vi "Servo Open comunication.vi"(8 "error in (no error)":errorcluster, 9 "IP address":T4) -> (0 "error out":errorcluster, 2 "Conections out":T3)   [LabVIEW 2017]
uses:
  <vilib>/addons/eal4LabVIEW/eal4LabVIEW.lvlib
  <vilib>/addons/eal4LabVIEW/ApiLib/Connection control/ealApiConnect_string.vi
  ctl/connections.ctl
  Servo drive module.lvlib
  ctl/Absolute actual position.ctl
  ctl/IP addresses.ctl
  ctl/Axis status.ctl
  ctl/Servo overall status.ctl
panel:
  in  "Overall status":T1
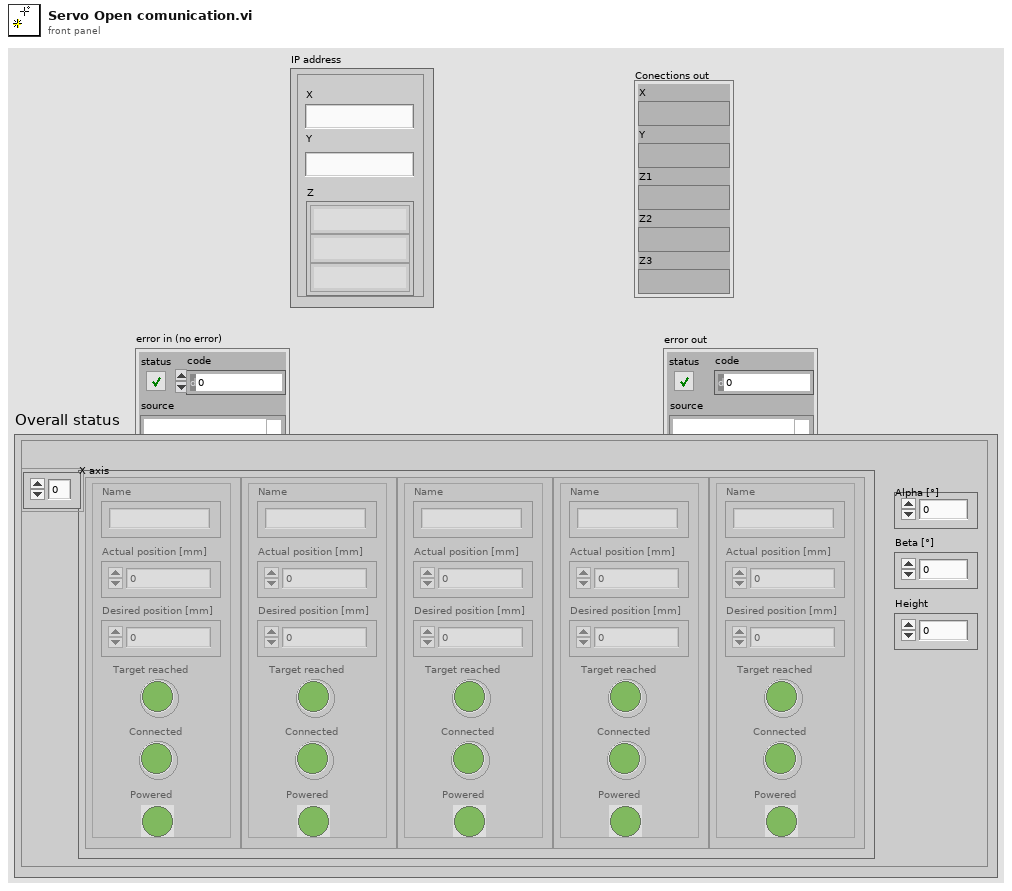
[diagram p1: front panel]
types:
  T1 = typedef "Servo drive module.lvlib/Servo overall status.ctl" = cluster{"X axis":T2[], "Alpha [°]":dbl, "Beta [°]":dbl, "Height":dbl}
  T2 = typedef "Servo drive module.lvlib/Axis status.ctl" = cluster{"Name":string, "Actual position [mm]":dbl, "Desired position [mm]":dbl, "Target reached":bool, "Connected":bool, "Powered":bool}
  T3 = typedef "Servo drive module.lvlib/connections.ctl" = cluster{"X":variant, "Y":variant, "Z1":variant, "Z2":variant, "Z3":variant}
  T4 = typedef "Servo drive module.lvlib/IP addresses.ctl" = cluster{"X":string, "Y":string, "Z":string[]}
  T5 = typedef "Servo drive module.lvlib/Absolute actual position.ctl" = cluster{"X":dbl, "Y":dbl, "Z1":dbl, "Z2":dbl, "Z3":dbl}
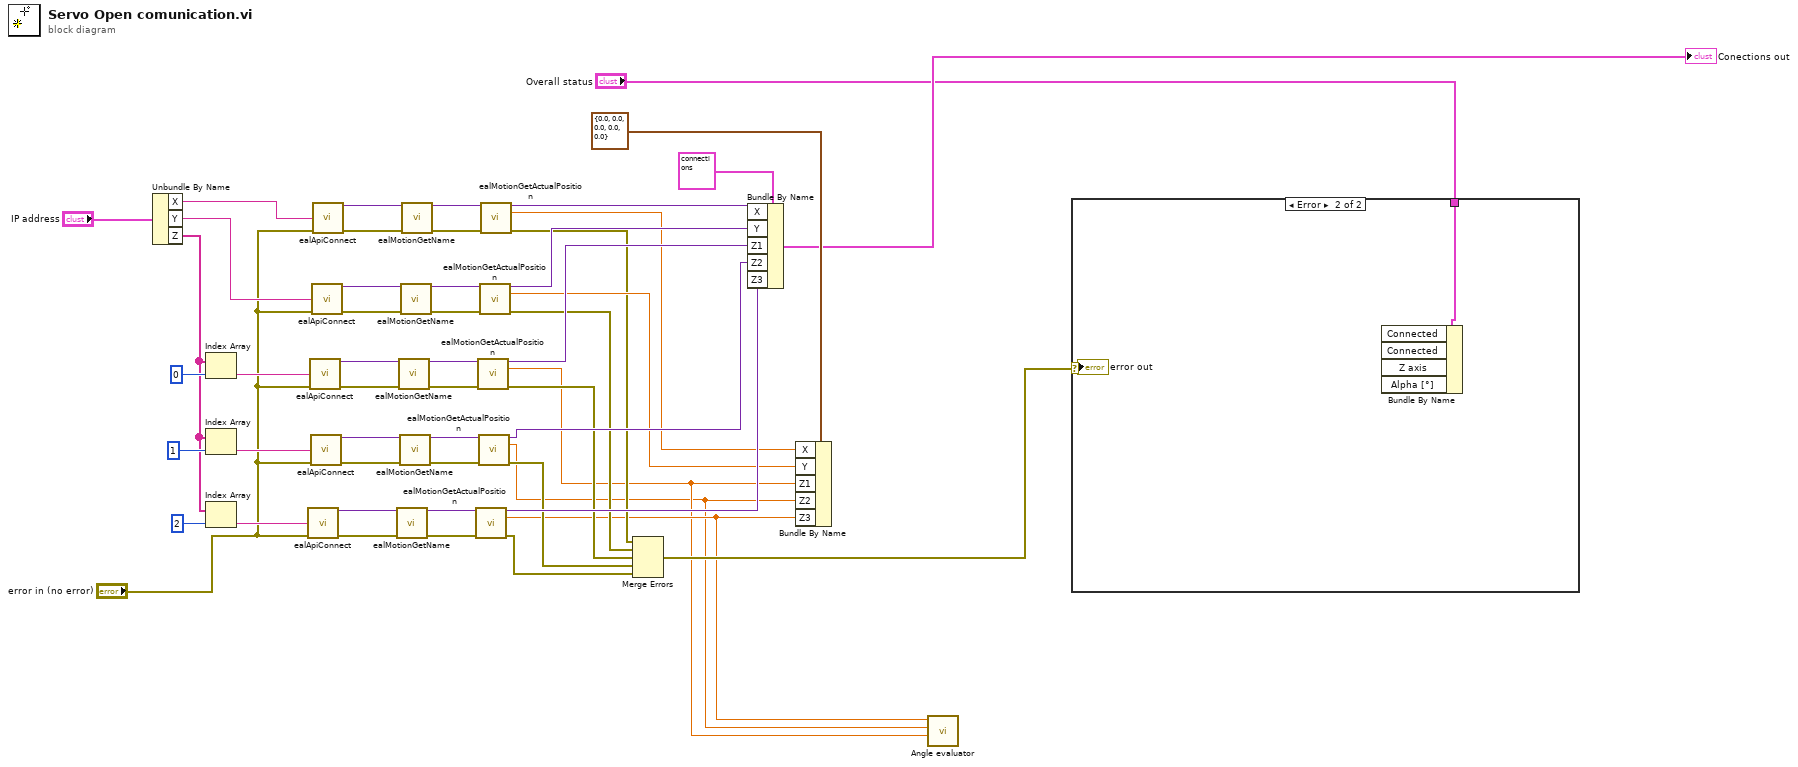
[diagram p0: block diagram]
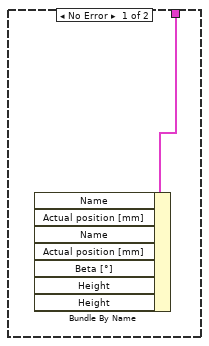
[diagram p2: hidden frame]
diagram:
  n1 = Unbundle By Name("IP address") -> ("X"=w43:string, "Y"=w44:string, "Z"=w45:string[])
  n2 = Index Array(array=w45, index=0) -> (element=w48:string)
  n3 = Index Array(array=w45, index=1) -> (element=w47:string)
  n4 = Index Array(array=w45, index=2) -> (element=w46:string)
  n5 = call-poly <vilib>:"ealApiConnect.vi"("ip address"=w46, "error in (no error)"="error in (no error)") -> ("connection out"=w29:variant, "error out"=w30:errorcluster)  [unwired: 12 in]
  n6 = call-poly <vilib>:"ealApiConnect.vi"("ip address"=w48, "error in (no error)"="error in (no error)") -> ("connection out"=w21:variant, "error out"=w22:errorcluster)  [unwired: 12 in]
  n7 = call-poly <vilib>:"ealApiConnect.vi"("ip address"=w47, "error in (no error)"="error in (no error)") -> ("connection out"=w26:variant, "error out"=w25:errorcluster)  [unwired: 12 in]
  n8 = call-poly <vilib>:"ealApiConnect.vi"("ip address"=w44, "error in (no error)"="error in (no error)") -> ("connection out"=w18:variant, "error out"=w17:errorcluster)  [unwired: 12 in]
  n9 = call-poly <vilib>:"ealApiConnect.vi"("ip address"=w43, "error in (no error)"="error in (no error)") -> ("connection out"=w13:variant, "error out"=w14:errorcluster)  [unwired: 12 in]
  n10 = call <vilib>:"ealMotionGetName.vi"("connection in"=w29, "error in (no error)"=w30) -> ("connection out"=w28:variant, "error out"=w31:errorcluster)  [unwired: 11 in, 1 out]
  n11 = call <vilib>:"ealMotionGetName.vi"("connection in"=w21, "error in (no error)"=w22) -> ("connection out"=w20:variant, "error out"=w23:errorcluster)  [unwired: 11 in, 1 out]
  n12 = call <vilib>:"ealMotionGetName.vi"("connection in"=w26, "error in (no error)"=w25) -> ("connection out"=w27:variant, "error out"=w24:errorcluster)  [unwired: 11 in, 1 out]
  n13 = call <vilib>:"ealMotionGetName.vi"("connection in"=w18, "error in (no error)"=w17) -> ("connection out"=w19:variant, "error out"=w16:errorcluster)  [unwired: 11 in, 1 out]
  n14 = call <vilib>:"ealMotionGetName.vi"("connection in"=w13, "error in (no error)"=w14) -> ("connection out"=w12:variant, "error out"=w15:errorcluster)  [unwired: 11 in, 1 out]
  n15 = call <vilib>:"ealMotionGetActualPosition.vi"("connection in"=w28, "error in (no error)"=w31) -> ("connection out"=w39:variant, "getActualPosition"=w3:dbl, "error out"=w7:errorcluster)  [unwired: 11 in]
  n16 = call <vilib>:"ealMotionGetActualPosition.vi"("connection in"=w20, "error in (no error)"=w23) -> ("connection out"=w37:variant, "getActualPosition"=w2:dbl, "error out"=w9:errorcluster)  [unwired: 11 in]
  n17 = call <vilib>:"ealMotionGetActualPosition.vi"("connection in"=w27, "error in (no error)"=w24) -> ("connection out"=w38:variant, "getActualPosition"=w1:dbl, "error out"=w8:errorcluster)  [unwired: 11 in]
  n18 = call <vilib>:"ealMotionGetActualPosition.vi"("connection in"=w19, "error in (no error)"=w16) -> ("connection out"=w36:variant, "getActualPosition"=w33:dbl, "error out"=w10:errorcluster)  [unwired: 11 in]
  n19 = call <vilib>:"ealMotionGetActualPosition.vi"("connection in"=w12, "error in (no error)"=w15) -> ("connection out"=w35:variant, "getActualPosition"=w32:dbl, "error out"=w11:errorcluster)  [unwired: 11 in]
  n20 = Merge Errors(w11, w10, w9, w8, w7) -> (w5:errorcluster)
  n21 = Bundle By Name(cluster=T3 {"X"=variant, "Y"=variant, "Z1"=variant, "Z2"=variant, "Z3"=variant} ("Conections in"), "X"=w35, "Y"=w36, "Z1"=w37, "Z2"=w38, "Z3"=w39) -> (→"Conections out":T3)
  n22 = Bundle By Name(cluster=T5 {"X"=0.0, "Y"=0.0, "Z1"=0.0, "Z2"=0.0, "Z3"=0.0} ("Actual position in"), "X"=w32, "Y"=w33, "Z1"=w2, "Z2"=w1, "Z3"=w3) -> ()  [unwired: 1 out]
  n23 = call "Angle evaluator.vi"("Position Az"=w2, "Position Bz"=w1, "Position Cz"=w3) -> ()  [unwired: 7 in, 2 out]
  n24 = case shown="Error" w5 {
    selector: w5 -> [_ w54]
    tunnel: "Overall status" -> [w52 w53]
    frame No Error {
      n25 = Bundle By Name(cluster=w52) -> ()  [unwired: 7 in, 1 out]
    }
    frame Error {
      n26 = Bundle By Name(cluster=w53) -> ()  [unwired: 4 in, 1 out]
      "error out" <- w54
    }
  }
